vi "Start Continuous Scan.vi"(8 "error in (no error)":errorcluster, 11 "NRT8000 in":refnum<class "NRT8000.lvclass">) -> (0 "error out":errorcluster, 3 "NRT8000 out":refnum<class "NRT8000.lvclass">)   [LabVIEW 2018, in "NRT8000.lvlib" / "NRT8000.lvclass"]
uses:
  NRT8000.lvclass
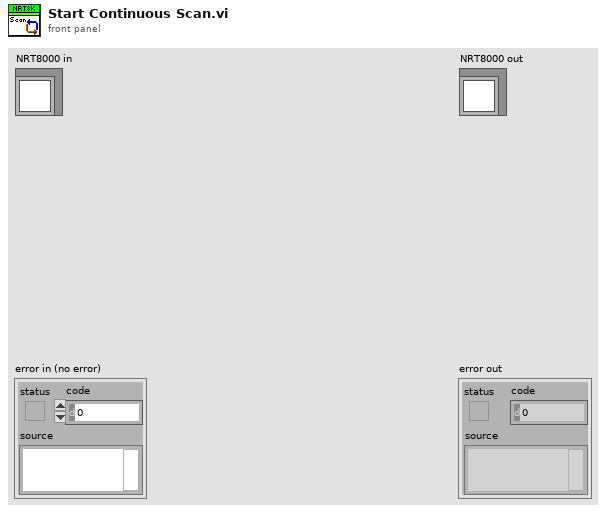
[diagram p1: front panel]
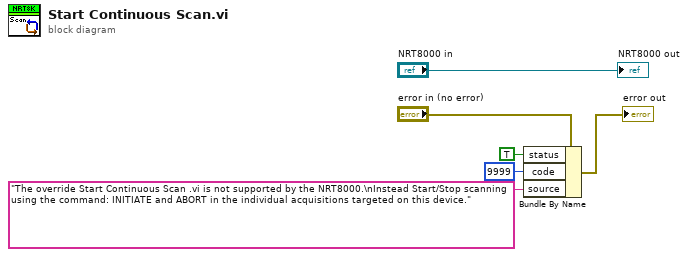
[diagram p0: block diagram]
diagram:
  n1 = Bundle By Name(cluster="error in (no error)", "status"=TRUE, "code"=9999, "source"="The override Start Continuous Scan .vi is not supported by the NRT8000.\nInstead Start/Stop scanning using the command: INITIATE and ABORT in the individual acquisitions targeted on this device.") -> (→"error out":errorcluster)
  "NRT8000 out" <- "NRT8000 in"
